vi "Ring Ref Get U16 String.vi"(8 "error in (no error)":errorcluster, 11 "Ring Ref U16":refnum<vi>) -> (0 "error out":errorcluster, 3 "Value string":string)   [LabVIEW 2018, in "Main Panel.lvlib" / "Main Panel.lvclass"]
uses:
  Main Panel.lvclass
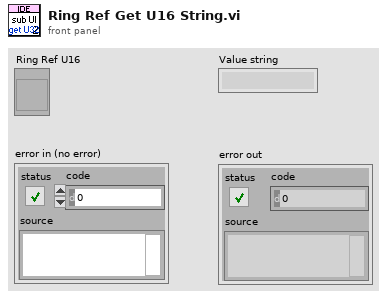
[diagram p1: front panel]
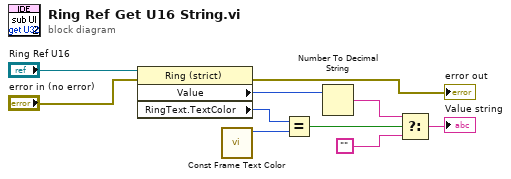
[diagram p0: block diagram]
diagram:
  n1 = property class="Ring (strict)"(reference="Ring Ref U16", error in="error in (no error)") -> (error out=→"error out":errorcluster, "Value"=w4:u16, "RingText.TextColor"=w2:u32)  [unwired: 1 out]
  n2 = call "Const Frame Text Color.vi"() -> ("valid num color"=w3:u32)  [unwired: 10 in, 1 out]
  n3 = Equal?(x=w2, y=w3) -> (x = y?=w1:bool)
  n4 = Number To Decimal String(number=w4) -> (decimal integer string=w8:string)  [unwired: 1 in]
  n5 = Select(t=w8, s=w1, f="") -> (s? t:f=→"Value string":string)
